vi "Display All Users In Manager.vi"(0 "User Manager View in":refnum<class "User Manager View.lvclass">, 5 "All Users In Manager":T1[](array[typedef]), 11 "error in (no error)":errorcluster) -> (4 "User Manager View out":refnum<class "User Manager View.lvclass">, 15 "error out":errorcluster)   [LabVIEW 2017, in "User Manager View.lvlib" / "User Manager View.lvclass"]
uses:
  <vilib>/gpm_packages/@cs/User Manager App/User Manager View/User Manager View/User Manager View.lvclass
  C:/Program Files/National Instruments/LabVIEW 2017/vi.lib/ActorFramework/Actor/Actor.lvclass
  <vilib>/gpm_packages/@cs/User Manager App/User Manager Model/Type Definitions/New User Information.ctl
  <vilib>/gpm_packages/@cs/User Manager App/User Manager Model/Type Definitions/Credentials.ctl
  <vilib>/gpm_packages/@cs/User Manager App/User Manager Model/Type Definitions/User Levels.ctl
  <vilib>/gpm_packages/@cs/User Manager App/User Manager View/User Manager Type Defs/State.ctl
  <vilib>/gpm_packages/@cs/User Manager App/User Manager View/User Manager View/User Manager View.lvclass/User Manager View.ctl
  <vilib>/ActorFramework/Actor/Actor.lvclass/Actor.ctl
  <vilib>/ActorFramework/Message Enqueuer/Message Enqueuer.lvclass/Message Enqueuer.ctl
  <vilib>/gpm_packages/@cs/User Manager App/User Manager View/User Manager View Messages/Pick User Msg/Pick User Msg.lvclass/Pick User Msg.ctl
  <vilib>/ActorFramework/Message Enqueuer/Init from Existing Queue.vi
  <vilib>/ActorFramework/Message Enqueuer/Enqueue.vi
  <vilib>/gpm_packages/@cs/User Manager App/User Manager View/User Manager View Messages/Pick User Msg/Pick User Msg.lvclass
  C:/Program Files/National Instruments/LabVIEW 2017/vi.lib/ActorFramework/Message/Message.lvclass
  <vilib>/ActorFramework/Message Priority Queue/Priority Enqueue.vi
  <vilib>/ActorFramework/Message Enqueuer/Message Enqueuer.lvclass
  <vilib>/gpm_packages/@cs/User Manager App/User Manager View/User Manager View.lvlib
  <vilib>/gpm_packages/@cs/User Manager App/User Manager Model/Type Definitions/User Manager Application Types.lvlib
  <vilib>/ActorFramework/Actor/Actor.lvclass
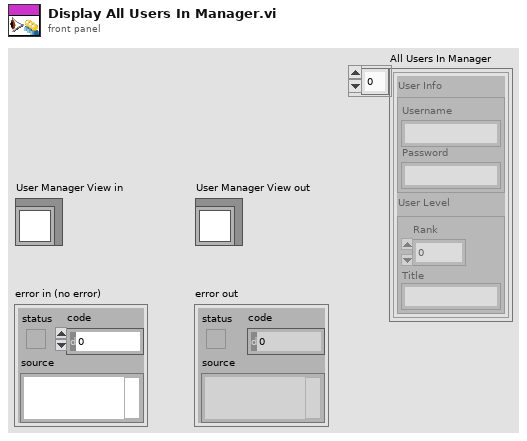
[diagram p1: front panel]
types:
  T1 = typedef "User Manager Application Types.lvlib/New User Information.ctl" = cluster{"User Info":T2, "User Level":T3}
  T2 = typedef "User Manager Application Types.lvlib/Credentials.ctl" = cluster{"Username":string, "Password":string}
  T3 = typedef "User Manager Application Types.lvlib/User Levels.ctl" = cluster{"Rank":i32, "Title":string}
  T4 = typedef "User Manager View.lvlib/State.ctl" = enum16{"Normal", "Adding User", "Changing User Data"}
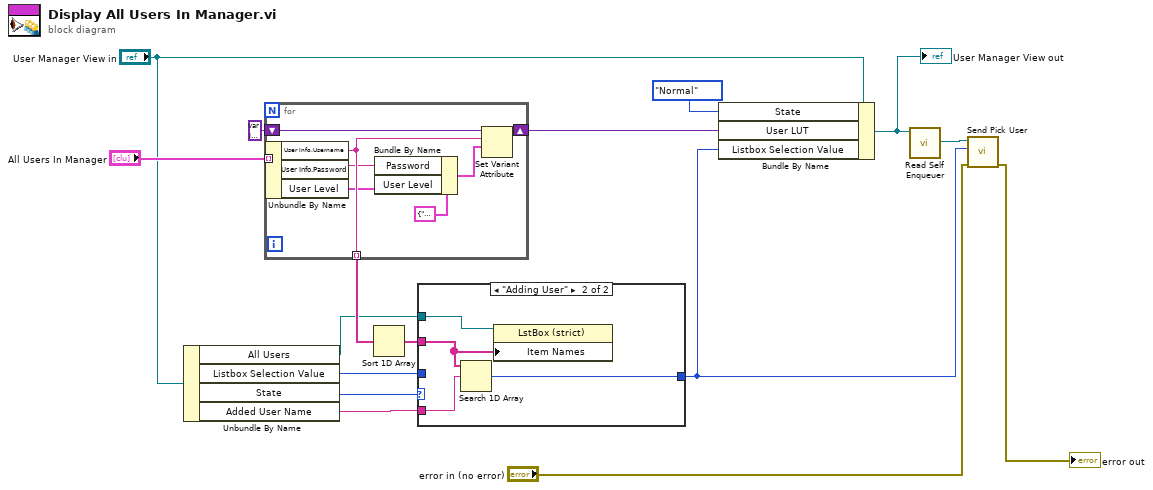
[diagram p0: block diagram]
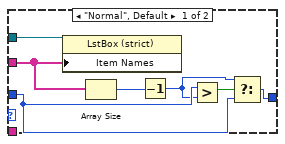
[diagram p2: hidden frame]
diagram:
  n1 = Unbundle By Name("User Manager View in") -> ("All Users"=w8:refnum<vi>, "Listbox Selection Value"=w9:i32, "State"=w12:T4, "Added User Name"=w11:string)
  n2 = for {
    tunnel: "All Users In Manager" -> [w22] mode=indexing
    shift-right: [w23] -> w14
    shift-left: variant -> [w24]
    tunnel: [w20] -> w15 mode=indexing
    n3 = Unbundle By Name(w22) -> ("User Info.Username"=w20:string, "User Info.Password"=w18:string, "User Level"=w19:T3)
    n4 = Bundle By Name(cluster=cluster{"Password":string, "User Level":T3} {"Password"="", "User Level"={"Rank"=0, "Title"=""}}, "Password"=w18, "User Level"=w19) -> (w21:cluster{"Password":string, "User Level":T3})
    n5 = Set Variant Attribute(Variant=w24, name=w20, value=w21) -> (Variant out=w23:variant)  [unwired: 1 in, 2 out]
  }
  n6 = Sort 1D Array(array=w15) -> (sorted array=w10:string[])
  n7 = case shown="\"Adding User\"" w12 {
    tunnel: w10 -> [w29 w34]
    tunnel: [w30 w32] -> w5
    tunnel: w11 -> [_ w33]
    tunnel: w8 -> [w28 w35]
    tunnel: w9 -> [w27 _]
    frame "Normal", Default {
      n8 = property class="LstBox (strict)"(reference=w28, "Item Names"=w29) -> ()  [unwired: 1 in, 2 out]
      n9 = Array Size(array=w29) -> (size(s)=w31:i32)
      n10 = Decrement(x=w31) -> (x-1=w26:i32)
      n11 = Greater?(x=w27, y=w26) -> (0:w25:bool)
      n12 = Select(t=w26, s=w25, f=w27) -> (s? t:f=w30:i32)
    }
    frame "Adding User" {
      n13 = Search 1D Array(1D array=w34, element=w33) -> (index of element=w32:i32)  [unwired: 1 in]
      n14 = property class="LstBox (strict)"(reference=w35, "Item Names"=w34) -> ()  [unwired: 1 in, 2 out]
    }
  }
  n15 = Bundle By Name(cluster="User Manager View in", "State"=State."Normal", "User LUT"=w14, "Listbox Selection Value"=w5) -> (w4:refnum<class "User Manager View.lvclass">)
  "User Manager View out" <- w4
  n16 = call <vilib>:"Read Self Enqueuer.vi"("Actor"=w4) -> ("Self Enqueuer"=w6:refnum<class "Message Enqueuer.lvclass">)  [unwired: 10 in]
  n17 = call <vilib>:"Send Pick User.vi"("error in (no error)"="error in (no error)", "NewVal"=w5, "Message Enqueuer"=w6) -> ("error out"=→"error out":errorcluster)  [unwired: 7 in, 1 out]
